vi "002_petlaZdarzen_MG.vi"() -> ()   [LabVIEW 2021]
panel:
  out "Kombinacja":u32
  out "Oczekiwanie":u32
  out "Czas start":u32
  out "Poprawana reakcja?":string="Tak"
  out "Czas reakcji [s]":dbl
  out "Prawa":bool=TRUE
  out "Lewa":bool
  in  "Start":bool
  in  "3":bool
  in  "2":bool
  in  "1":bool
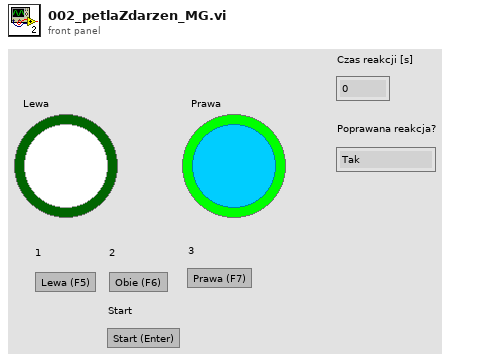
[diagram p1: front panel]
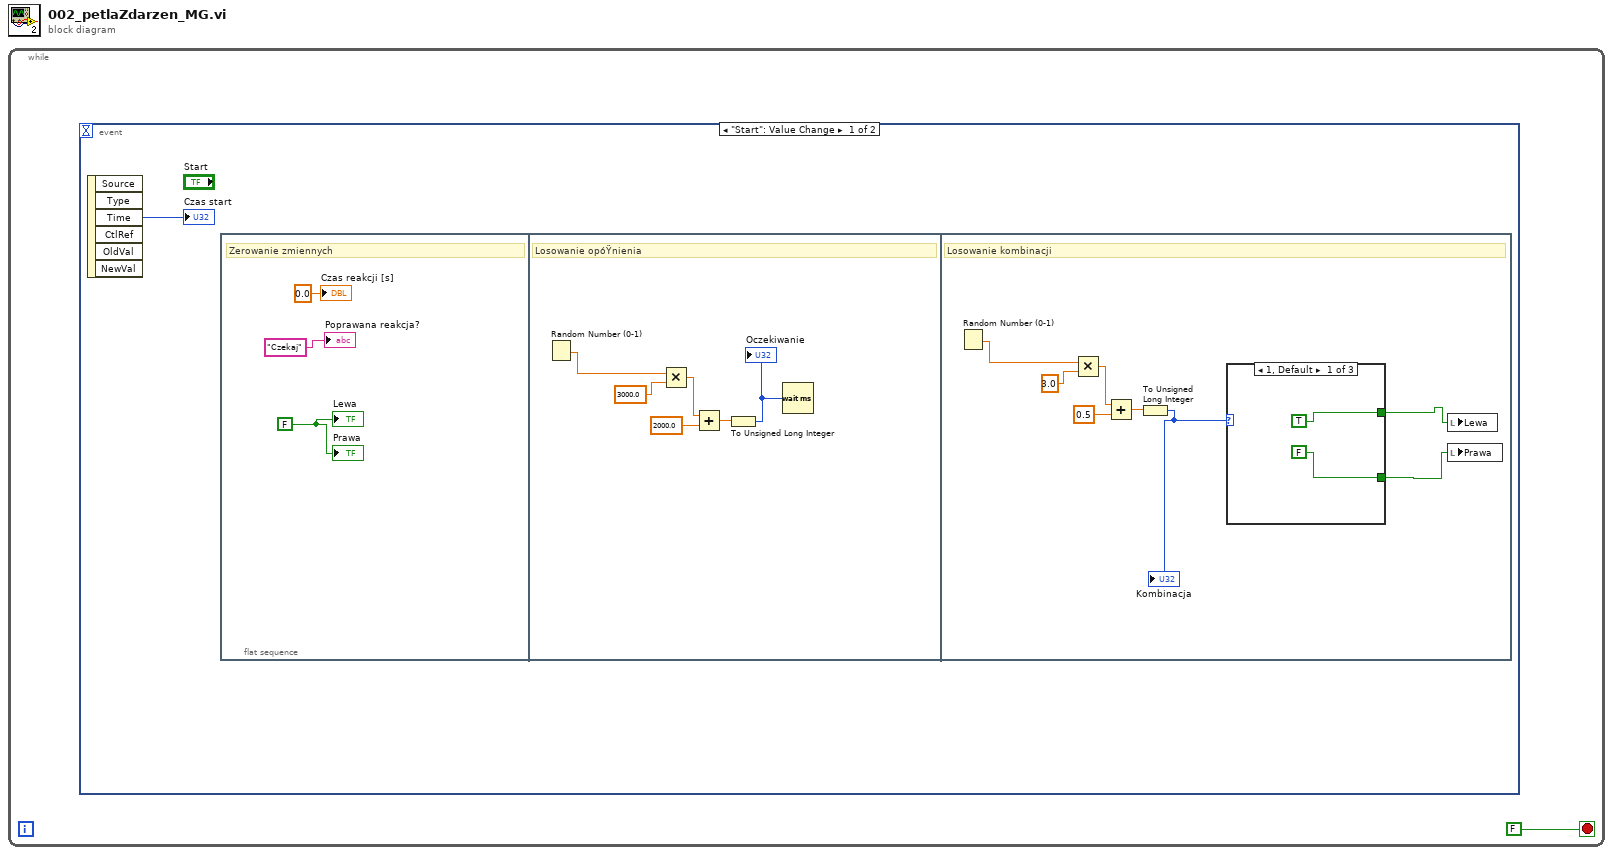
[diagram p0: block diagram]
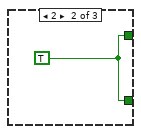
[diagram p2: hidden frame]
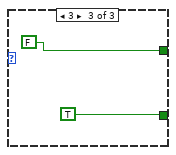
[diagram p3: hidden frame]
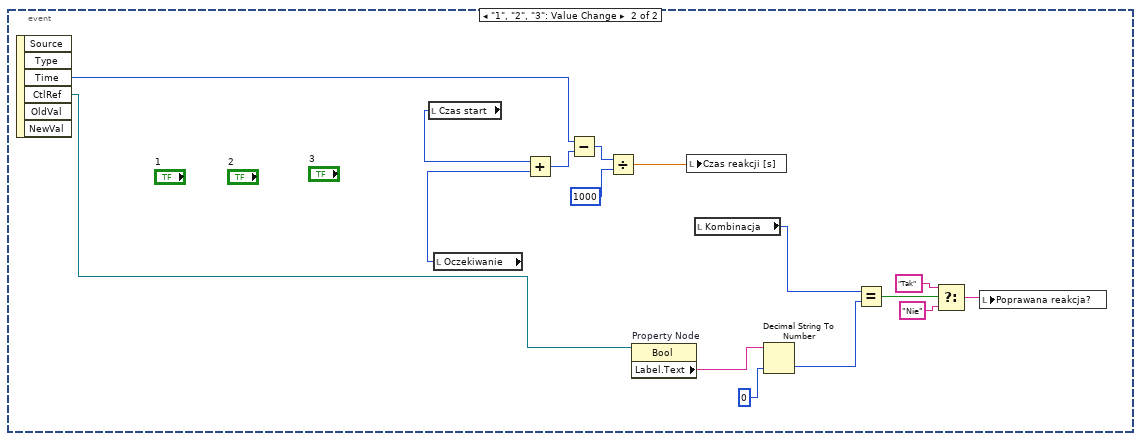
[diagram p4: hidden frame]
diagram:
  n1 = while {
    stop <- FALSE stop-if-true
    n2 = event shown="[0] \"Start\": Value Change" {
      selector: _ -> [_ _]
      dyn-events: _ -> [_ _]
      timeout: _ -> [_ _]
      event "Start": Value Change {
        n3 = event-data() -> ("Time"=→"Czas start":u32)  [unwired: 1 in, 5 out]
        n4 = flat-sequence {
          frame #0 {
            w3 = FALSE ("Lewa")
            # "Zerowanie zmiennych"
            "Poprawana reakcja?" <- "Czekaj" ("Poprawana reakcja?")
            "Czas reakcji [s]" <- 0.0 ("Czas reakcji [s]")
            "Lewa" <- w3
            "Prawa" <- w3
          }
          frame #1 {
            # "Losowanie opóŸnienia"
            n5 = Random Number (0-1)() -> (number: 0 to 1=w11:dbl)
            n6 = Multiply(x=w11, y=3000.0) -> (x*y=w9:dbl)
            n7 = Add(x=w9, y=2000.0) -> (x+y=w7:dbl)
            n8 = To Unsigned Long Integer(number=w7) -> (unsigned 32bit integer=w6:u32)
            "Oczekiwanie" <- w6
            n9 = Wait (ms)(milliseconds to wait=w6) -> ()  [unwired: 1 out]
          }
          frame #2 {
            # "Losowanie kombinacji"
            n10 = Random Number (0-1)() -> (number: 0 to 1=w19:dbl)
            n11 = Multiply(x=w19, y=3.0) -> (x*y=w17:dbl)
            n12 = Add(x=w17, y=0.5) -> (x+y=w15:dbl)
            n13 = To Unsigned Long Integer(number=w15) -> (unsigned 32bit integer=w14:u32)
            "Kombinacja" <- w14
            n14 = case shown="1, Default" w14 {
              tunnel: [TRUE w22 FALSE] -> w13
              tunnel: [FALSE w22 TRUE] -> w12
              frame 1, Default {
              }
              frame 2 {
                w22 = TRUE
              }
              frame 3 {
              }
            }
            n15 = local write "Lewa"(w13) -> ()
            n16 = local write "Prawa"(w12) -> ()
          }
        }
      }
      event "1", "2", "3": Value Change {
        n17 = event-data() -> ("Time"=w37:u32, "CtlRef"=w33:refnum<vi>)  [unwired: 1 in, 4 out]
        n18 = local read "Czas start"() -> (w39:u32)
        n19 = local read "Oczekiwanie"() -> (w38:u32)
        n20 = Add(x=w39, y=w38) -> (x+y=w40:u32)
        n21 = Subtract(x=w37, y=w40) -> (x-y=w36:u32)
        n22 = Divide(x=w36, y=u32 1000) -> (x/y=w34:dbl)
        n23 = property on="Property Node" class="Bool"(reference=w33) -> ("Label.Text"=w32:string)  [unwired: 1 in, 2 out]
        n24 = local write "Czas reakcji [s]"(w34) -> ()
        n25 = local read "Kombinacja"() -> (w29:u32)
        n26 = Decimal String To Number(string=w32, default (0L)=u8 0 ("default (0 I32)")) -> (number=w30:u8)  [unwired: 1 in, 1 out]
        n27 = Equal?(x=w29, y=w30) -> (x = y?=w28:bool)
        n28 = Select(t="Tak", s=w28, f="Nie") -> (s? t:f=w25:string)
        n29 = local write "Poprawana reakcja?"(w25) -> ()
      }
    }
  }
